vi "Ball Vision Align.vi"(10 "Dashboard Drivetrain Command":T3, 11 "Ball Vision Packet":T1) -> (2 "Aligned?":bool, 3 "Turn Power":dbl)   [LabVIEW 2015]
uses:
  Common Code/Dashboard Drivetrain Command.ctl
  Common Code/Drivetrain Vision.ctl
  Common Code/Ball Vision Packet.ctl
  Common Code/Tracking Mode.ctl
  <vilib>/addons/control/pid/NI_PID_pid.lvlib
  <vilib>/addons/control/pid/pid.llb/PID (DBL).vi
panel:
  in  "Changed?":bool
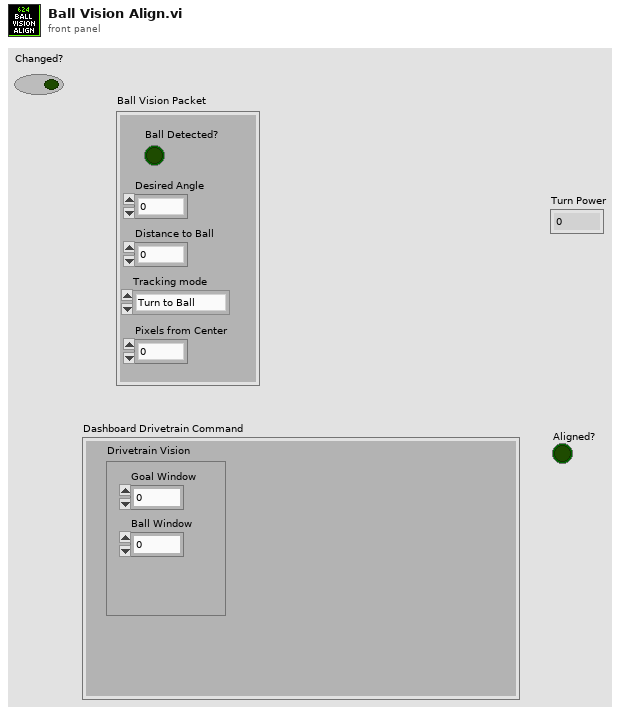
[diagram p1: front panel]
types:
  T1 = typedef "Ball Vision Packet.ctl" = cluster{"Ball Detected?":bool, "Distance to Ball":dbl, "Desired Angle":dbl, "Pixels from Center":dbl, "Tracking mode":T2}
  T2 = typedef "Tracking Mode.ctl" = enum16{"Turn to Ball", "Turn to Angle"}
  T3 = typedef "Dashboard Drivetrain Command.ctl" = cluster{"Drivetrain Vision":T4}
  T4 = typedef "Drivetrain Vision.ctl" = cluster{"Goal Window":dbl, "Ball Window":dbl}
  T5 = cluster{"proportional gain (Kc)":dbl, "integral time (Ti, min)":dbl, "derivative time (Td, min)":dbl}
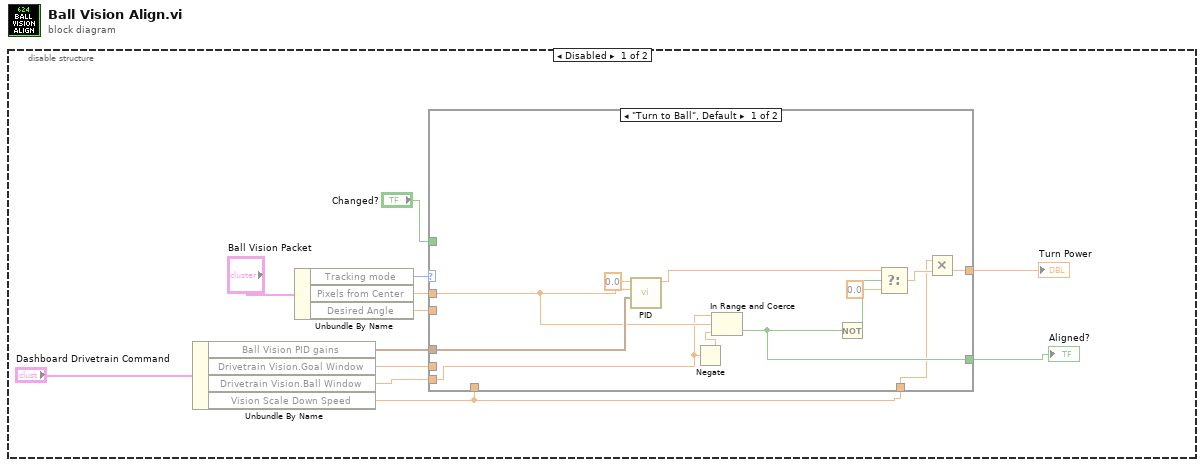
[diagram p0: block diagram]
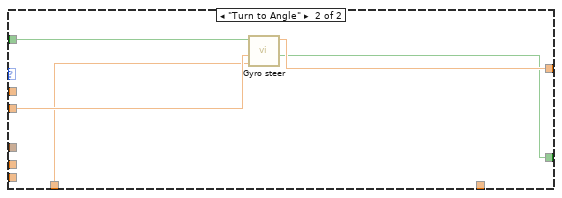
[diagram p2: hidden frame]
diagram:
  n1 = disable-structure shown="Disabled" {
    frame Disabled {
      n2 = Unbundle By Name("Dashboard Drivetrain Command") -> ("Ball Vision PID gains"=w8:T5, "Drivetrain Vision.Goal Window"=w6:dbl, "Drivetrain Vision.Ball Window"=w5:dbl, "Vision Scale Down Speed"=w2:dbl)
      n3 = Unbundle By Name("Ball Vision Packet") -> ("Tracking mode"=w10:T2, "Pixels from Center"=w9:dbl, "Desired Angle"=w3:dbl)
      n4 = case shown="\"Turn to Ball\", Default" w10 {
        tunnel: w9 -> [w21 _]
        tunnel: w8 -> [w24 _]
        tunnel: [w16 w27] -> w7
        tunnel: w6 -> [_ _]
        tunnel: w5 -> [w13 _]
        tunnel: w2 -> [w15 _]
        tunnel: [w19 w26] -> w4
        tunnel: w3 -> [_ w29]
        tunnel: w2 -> [_ w28]
        tunnel: "Changed?" -> [_ w25]
        frame "Turn to Ball", Default {
          n5 = call-poly <vilib>:"PID.vi"("PID gains"=w24, "process variable"=w21, "setpoint"=0.0) -> ("output"=w22:dbl)  [unwired: 7 in, 1 out]
          n6 = Negate(x=w13) -> (-x=w14:dbl)
          n7 = In Range and Coerce(upper limit=w13, x=w21, lower limit=w14) -> (In Range?=w19:bool)  [unwired: 1 out]
          n8 = Not(x=w19) -> (.not. x?=w18:bool)
          n9 = Select(t=w22, s=w18, f=0.0) -> (s? t:f=w17:dbl)
          n10 = Multiply(x=w15, y=w17) -> (x*y=w16:dbl)
        }
        frame "Turn to Angle" {
          n11 = call "Gyro steer.vi"("Turn Speed"=w28, "Target Angle"=w29, "Changed?"=w25) -> ("In Range?"=w26:bool, "X out"=w27:dbl)  [unwired: 7 in]
        }
      }
      "Turn Power" <- w7
      "Aligned?" <- w4
    }
    frame Enabled {
    }
  }
